vi "Test Stop.vi"(11 "Error in":errorcluster) -> (15 "Error out":errorcluster)   [LabVIEW 2020, in "StopWatchTests.lvlib"]
doc: "This VI validates the stop button"
uses:
  StopWatchTests.lvlib
  <vilib>/SLL Drona/APIs/Assert/AssertVI/AssertVIExecRunning.vi
  <vilib>/SLL Drona/APIs/Stimulus/ControlValue/SetValueAuto.vi
  <vilib>/SLL Drona/APIs/Assert/AssertVI/AssertVIExecIdle.vi
  <vilib>/SLL Drona/APIs/Stimulus/VI/CloseVI.vi
  <vilib>/SLL Drona/Drona.lvlib
  <vilib>/addons/_JKI Toolkits/Caraya/classes/Test/Test.lvclass
  <vilib>/SLL Drona/APIs/Assert/AssertVI/AssertVI.lvlib
  <vilib>/SLL Drona/APIs/Stimulus/ControlValue/ControlValue.lvlib
  <vilib>/SLL Drona/APIs/Stimulus/VI/VI.lvlib
  <vilib>/Wiresmith Technology/G CLI/CLI Class/CLI.lvclass
panel:
  # "STOP TEST"
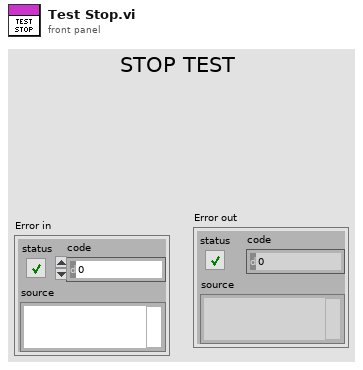
[diagram p1: front panel]
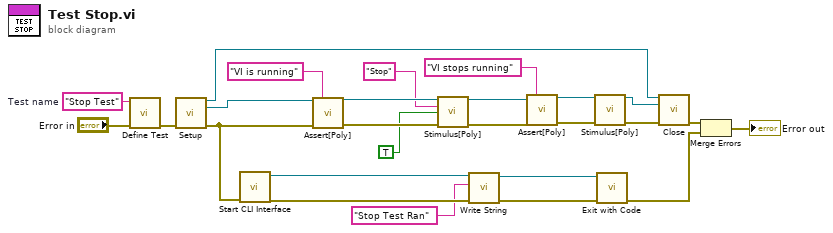
[diagram p0: block diagram]
diagram:
  w24 = "Stop Test"  # Test name
  n1 = call <vilib>:"Define Test.vi"("error in (no error)"="Error in", "Label (VI Title)"=w24) -> ("error out"=w25:errorcluster)  [unwired: 9 in]
  n2 = call <vilib>:"Setup.vi"("error in"=w25) -> ("Application Ref"=w23:refnum<vi>, "VI Reference Out"=w19:refnum<vi>, "error out"=w9:errorcluster)  [unwired: 12 in]
  n3 = call <vilib>:"Start CLI Interface.vi"("error in (no error)"=w9) -> ("error out"=w8:errorcluster, "CLI out"=w7:refnum<class "CLI.lvclass">)  [unwired: 7 in, 2 out]
  n4 = call-poly <vilib>:"Assert[Poly].vi"("VI Reference In"=w19, "Test Label"="VI is running", "Error In"=w9) -> ("VI Reference Out"=w17:refnum<vi>, "Error Out"=w18:errorcluster)  [unwired: 11 in]
  n5 = call-poly <vilib>:"Stimulus[Poly].vi"("VI Reference In"=w17, "Control Path"="Stop", "Value (Signaling)"=TRUE, "error in"=w18) -> ("VI Reference Out"=w13:refnum<vi>, "error out"=w14:errorcluster)  [unwired: 10 in]
  n6 = call <vilib>:"Write String.vi"("error in (no error)"=w8, "Text to Write"="Stop Test Ran", "CLI in"=w7) -> ("error out"=w5:errorcluster, "CLI out"=w4:refnum<class "CLI.lvclass">)  [unwired: 7 in]
  n7 = call-poly <vilib>:"Assert[Poly].vi"("VI Reference In"=w13, "Test Label"="VI stops running", "Error In"=w14) -> ("VI Reference Out"=w10:refnum<vi>, "Error Out"=w11:errorcluster)  [unwired: 11 in]
  n8 = call-poly <vilib>:"Stimulus[Poly].vi"("VI Reference In"=w10, "error in"=w11) -> ("VI Reference Out"=w22:refnum<vi>, "error out"=w21:errorcluster)  [unwired: 12 in]
  n9 = call <vilib>:"Exit with Code.vi"("error in (no error)"=w5, "CLI in"=w4) -> ("error out"=w2:errorcluster)  [unwired: 9 in]
  n10 = call <vilib>:"Close.vi"("Application Ref"=w23, "VI Reference"=w22, "error in"=w21) -> ("error out"=w3:errorcluster)  [unwired: 12 in]
  n11 = Merge Errors(w3, w2) -> (→"Error out":errorcluster)
